vi "Get applicable selectors.vi"(8 "Error in":errorcluster, 11 "GObject":refnum<vi>) -> (0 "Error out":errorcluster, 3 "Selectors":string[](array[string]))   [LabVIEW 2019, in "LSS.lvlib"]
doc: "This recursive function is used to obtain all LSS selectors that could apply to a given object. For example, a reference to a boolean control on a normal front panel would return the name of the boolean, the class boolean, and the panel. \n\n<b>Inputs:</b>\n<b>GObject</b> - Reference to the UI object for which this VI will find selectors.\n<b>Error In</b> - Error input terminal\n\n<b>Outputs:</b>\n<b>Selectors</b> - List of applicable selectors for the GObject reference input.\n<b>Error Out</b> - Error output terminal"
uses:
  LSS.lvlib
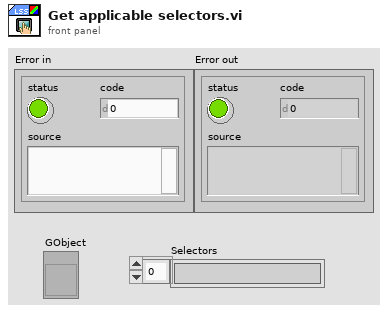
[diagram p1: front panel]
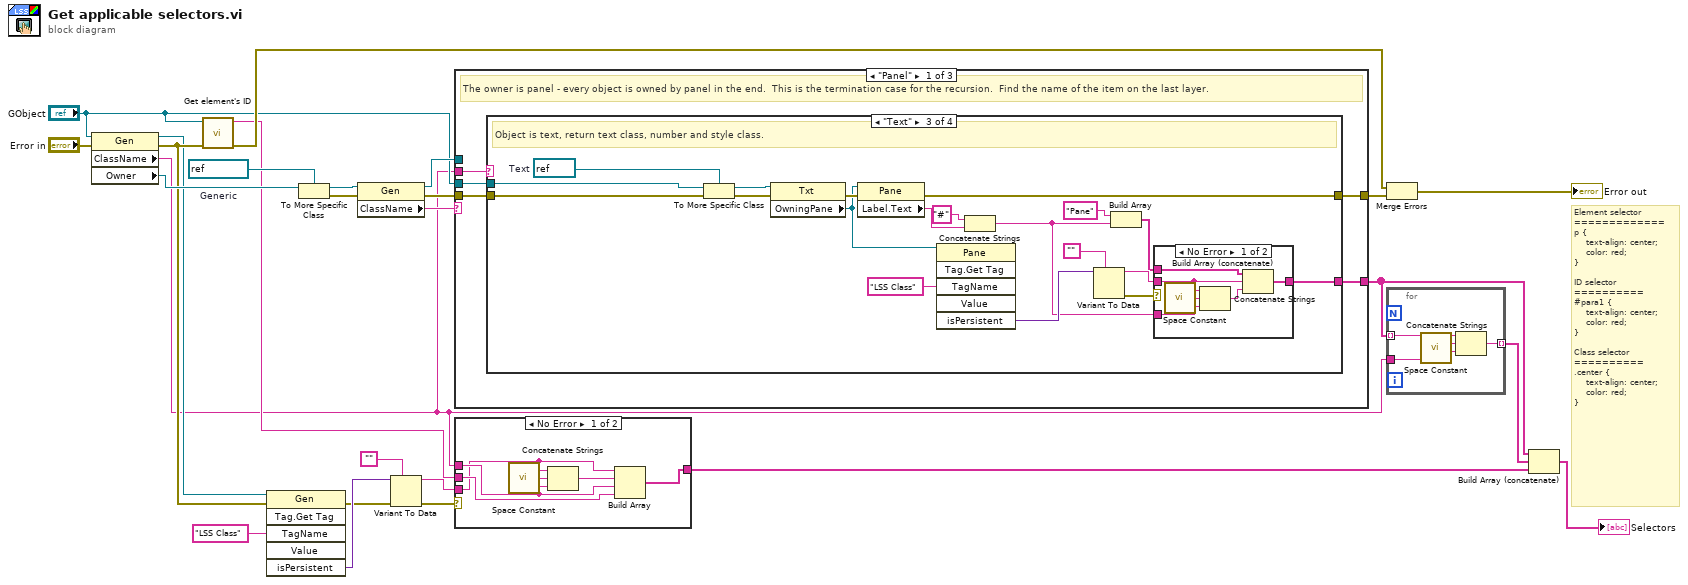
[diagram p0: block diagram]
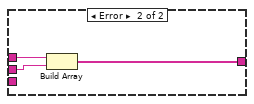
[diagram p2: hidden frame]
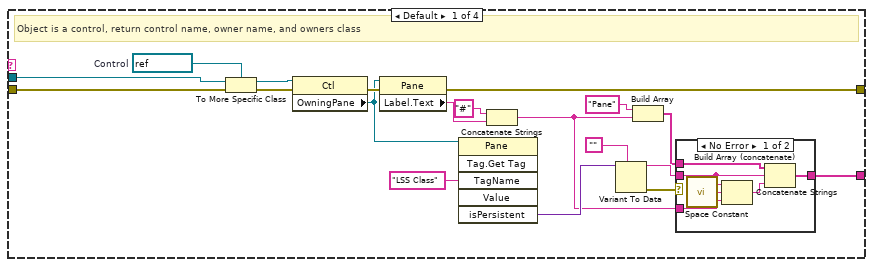
[diagram p3: hidden frame]
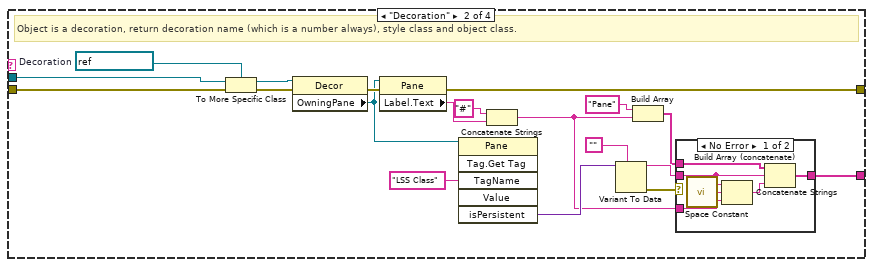
[diagram p5: hidden frame]
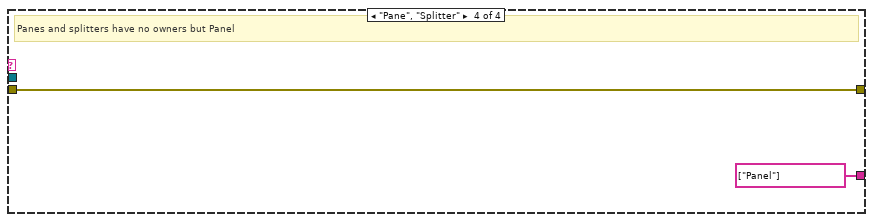
[diagram p8: hidden frame]
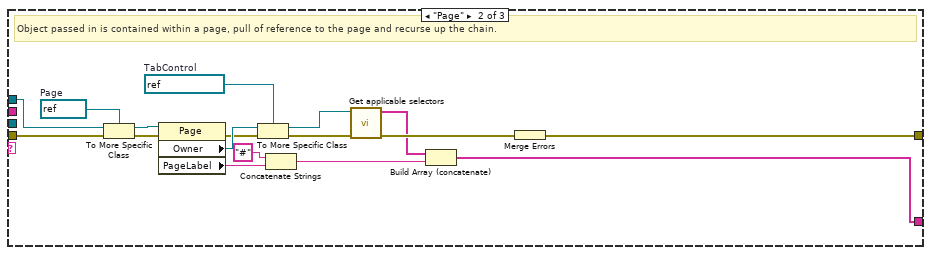
[diagram p9: hidden frame]
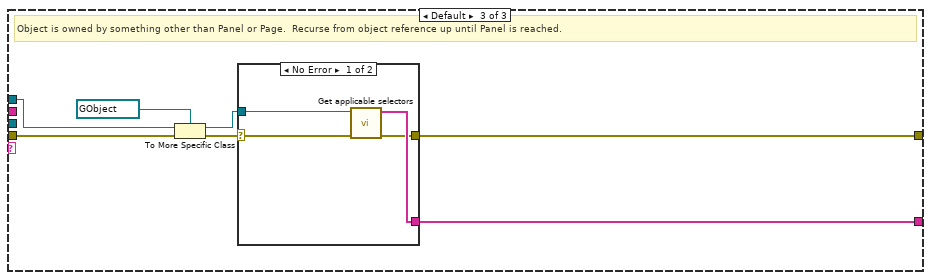
[diagram p10: hidden frame]
diagram:
  w22 = refnum<vi> refnum  # Generic
  # "Element selector\n=============\np {\n    text-align: center;\n    color: red;\n}\n\nID selector\n==========\n#para1 {\n    text-align: center;\n    color: red;\n}\n\nClass selector\n==========\n.center {\n    text-align: center;\n    color: red;\n}"
  n1 = property class="Gen"(reference="GObject", error in="Error in") -> (reference out=w7:refnum<vi>, error out=w19:errorcluster, "ClassName"=w2:string, "Owner"=w23:refnum<vi>)
  n2 = call "Get element's ID.vi"("Error in"=w19, "GObject in"="GObject") -> ("Error out"=w18:errorcluster, "ID"=w8:string)  [unwired: 8 in]
  n3 = invoke class="Gen" method="Tag.Get Tag"(reference=w7, error in=w19, "TagName"="LSS Class" ("Tag Name")) -> (error out=w17:errorcluster, "isPersistent"=w25:variant)  [unwired: 3 in, 4 out]
  n4 = To More Specific Class(target class=w22, reference=w23) -> (specific class reference=w13:refnum<vi>, error out=w21:errorcluster)  [unwired: 1 in]
  n5 = property class="Gen"(reference=w13, error in=w21) -> (reference out=w12:refnum<vi>, error out=w14:errorcluster, "ClassName"=w5:string)
  n6 = Variant To Data(error in=w17, type="", Variant=w25) -> (data=w10:string, error out=w11:errorcluster)
  n7 = case shown="\"Panel\"" w5 {
    tunnel: [w29 w121 w135] -> w1
    tunnel: [w27 w128 w134] -> w16
    tunnel: w14 -> [w28 w118 w130]
    tunnel: w12 -> [_ w127 w133]
    tunnel: "GObject" -> [w31 _ _]
    tunnel: w2 -> [w30 _ _]
    frame "Panel" {
      # "The owner is panel - every object is owned by panel in the end.  This is the termination case for the recursion.  Find the name of the item on the last layer."
      n8 = case shown="\"Text\"" w30 {
        tunnel: w31 -> [w42 w69 w95 _]
        tunnel: [w33 w60 w86 string[] ["Panel"]] -> w29
        tunnel: w28 -> [w46 w73 w99 w110]
        tunnel: [w43 w70 w96 w110] -> w27
        frame Default {
          w50 = refnum<vi> refnum  # Control
          # "Object is a control, return control name, owner name, and owners class"
          n9 = To More Specific Class(target class=w50, reference=w42, error in=w46) -> (specific class reference=w49:refnum<vi>, error out=w45:errorcluster)
          n10 = property class="Ctl"(reference=w49, error in=w45) -> (error out=w44:errorcluster, "OwningPane"=w39:refnum<vi>)  [unwired: 1 out]
          n11 = property class="Pane"(reference=w39, error in=w44) -> (error out=w43:errorcluster, "Label.Text"=w48:string)  [unwired: 1 out]
          n12 = invoke class="Pane" method="Tag.Get Tag"(reference=w39, "TagName"="LSS Class" ("Tag Name")) -> ("isPersistent"=w37:variant)  [unwired: 4 in, 5 out]
          n13 = Concatenate Strings("#" ("string"), w48) -> (w32:string)
          n14 = Variant To Data(type="", Variant=w37) -> (data=w35:string, error out=w36:errorcluster)  [unwired: 1 in]
          n15 = Build Array("Pane" ("element"), w32) -> (w34:string[])
          n16 = case shown="No Error" w36 {
            tunnel: w35 -> [w53 _]
            tunnel: w34 -> [w55 w57]
            tunnel: [w56 w57] -> w33
            tunnel: w32 -> [w51 _]
            frame No Error {
              n17 = call <vilib>:"Space Constant.vi"() -> ("String"=w54:string)
              n18 = Concatenate Strings(w53, w54, w51) -> (w52:string)
              n19 = Build Array (concatenate)(w55, w53, w52) -> (w56:string[])
            }
            frame Error {
            }
          }
        }
        frame "Decoration" {
          w58 = refnum<vi> refnum  # Decoration
          # "Object is a decoration, return decoration name (which is a number always), style class and object class."
          n20 = To More Specific Class(target class=w58, reference=w69, error in=w73) -> (specific class reference=w76:refnum<vi>, error out=w72:errorcluster)
          n21 = property class="Decor"(reference=w76, error in=w72) -> (error out=w71:errorcluster, "OwningPane"=w66:refnum<vi>)  [unwired: 1 out]
          n22 = property class="Pane"(reference=w66, error in=w71) -> (error out=w70:errorcluster, "Label.Text"=w75:string)  [unwired: 1 out]
          n23 = invoke class="Pane" method="Tag.Get Tag"(reference=w66, "TagName"="LSS Class" ("Tag Name")) -> ("isPersistent"=w64:variant)  [unwired: 4 in, 5 out]
          n24 = Concatenate Strings("#" ("string"), w75) -> (w59:string)
          n25 = Variant To Data(type="", Variant=w64) -> (data=w62:string, error out=w63:errorcluster)  [unwired: 1 in]
          n26 = Build Array("Pane" ("element"), w59) -> (w61:string[])
          n27 = case shown="No Error" w63 {
            tunnel: w62 -> [w79 _]
            tunnel: w61 -> [w81 w83]
            tunnel: [w82 w83] -> w60
            tunnel: w59 -> [w77 _]
            frame No Error {
              n28 = call <vilib>:"Space Constant.vi"() -> ("String"=w80:string)
              n29 = Concatenate Strings(w79, w80, w77) -> (w78:string)
              n30 = Build Array (concatenate)(w81, w79, w78) -> (w82:string[])
            }
            frame Error {
            }
          }
        }
        frame "Text" {
          w84 = refnum<vi> refnum  # Text
          # "Object is text, return text class, number and style class."
          n31 = To More Specific Class(target class=w84, reference=w95, error in=w99) -> (specific class reference=w102:refnum<vi>, error out=w98:errorcluster)
          n32 = property class="Txt"(reference=w102, error in=w98) -> (error out=w97:errorcluster, "OwningPane"=w92:refnum<vi>)  [unwired: 1 out]
          n33 = property class="Pane"(reference=w92, error in=w97) -> (error out=w96:errorcluster, "Label.Text"=w101:string)  [unwired: 1 out]
          n34 = invoke class="Pane" method="Tag.Get Tag"(reference=w92, "TagName"="LSS Class" ("Tag Name")) -> ("isPersistent"=w90:variant)  [unwired: 4 in, 5 out]
          n35 = Concatenate Strings("#" ("string"), w101) -> (w85:string)
          n36 = Variant To Data(type="", Variant=w90) -> (data=w88:string, error out=w89:errorcluster)  [unwired: 1 in]
          n37 = Build Array("Pane" ("element"), w85) -> (w87:string[])
          n38 = case shown="No Error" w89 {
            tunnel: w88 -> [w105 _]
            tunnel: w87 -> [w107 w109]
            tunnel: [w108 w109] -> w86
            tunnel: w85 -> [w103 _]
            frame No Error {
              n39 = call <vilib>:"Space Constant.vi"() -> ("String"=w106:string)
              n40 = Concatenate Strings(w105, w106, w103) -> (w104:string)
              n41 = Build Array (concatenate)(w107, w105, w104) -> (w108:string[])
            }
            frame Error {
            }
          }
        }
        frame "Pane", "Splitter" {
          # "Panes and splitters have no owners but Panel"
        }
      }
    }
    frame "Page" {
      w124 = refnum<vi> refnum  # TabControl
      w126 = refnum<vi> refnum  # Page
      # "Object passed in is contained within a page, pull of reference to the page and recurse up the chain."
      n42 = To More Specific Class(target class=w126, reference=w127, error in=w118) -> (specific class reference=w125:refnum<vi>, error out=w117:errorcluster)
      n43 = property class="Page"(reference=w125, error in=w117) -> (error out=w116:errorcluster, "Owner"=w123:refnum<vi>, "PageLabel"=w119:string)  [unwired: 1 out]
      n44 = To More Specific Class(target class=w124, reference=w123, error in=w116) -> (specific class reference=w122:refnum<vi>, error out=w115:errorcluster)
      n45 = Concatenate Strings("#" ("string"), w119) -> (w112:string)
      n46 = call "Get applicable selectors.vi"("Error in"=w115, "GObject"=w122) -> ("Error out"=w114:errorcluster, "Selectors"=w113:string[])  [unwired: 8 in]
      n47 = Build Array (concatenate)(w113, w112) -> (w121:string[])
      n48 = Merge Errors(w114) -> (w128:errorcluster)
    }
    frame Default {
      # "Object is owned by something other than Panel or Page.  Recurse from object reference up until Panel is reached."
      n49 = To More Specific Class(target class=refnum<vi> refnum, reference=w133, error in=w130) -> (specific class reference=w132:refnum<vi>, error out=w129:errorcluster)
      n50 = case shown="No Error" w129 {
        selector: w129 -> [w137 w140]
        tunnel: [w139 _] -> w135
        tunnel: w132 -> [w138 _]
        tunnel: [w136 w140] -> w134
        frame No Error {
          n51 = call "Get applicable selectors.vi"("Error in"=w137, "GObject"=w138) -> ("Error out"=w136:errorcluster, "Selectors"=w139:string[])  [unwired: 8 in]
        }
        frame Error {
        }
      }
    }
  }
  n52 = case shown="No Error" w11 {
    tunnel: w8 -> [w144 w149]
    tunnel: w10 -> [w141 _]
    tunnel: [w146 w148] -> w9
    tunnel: w2 -> [w143 w147]
    frame No Error {
      n53 = call <vilib>:"Space Constant.vi"() -> ("String"=w145:string)
      n54 = Concatenate Strings(w141, w145, w143) -> (w142:string)
      n55 = Build Array(w141, w142, w143, w144) -> (w146:string[])
    }
    frame Error {
      n56 = Build Array(w147, w149) -> (w148:string[])
    }
  }
  n57 = Merge Errors(w18, w16) -> (→"Error out":errorcluster)
  n58 = for {
    tunnel: w1 -> [w151] mode=indexing
    tunnel: w2 -> [w150]
    tunnel: [w153] -> w3 mode=indexing
    n59 = call <vilib>:"Space Constant.vi"() -> ("String"=w152:string)
    n60 = Concatenate Strings(w151, w152, w150) -> (w153:string)
  }
  n61 = Build Array (concatenate)(w1, w3, w9) -> (→"Selectors":string[])
